vi "rx QAM.vi"() -> ()   [LabVIEW 2026]
uses:
  <instrlib>/niUSRP/niUSRP Fetch Rx Data (CDB Cluster).vi
  <vilib>/addons/Modulation/Digital/Demodulation/MT Calculate BER After Trigger (User Pattern).vi
  <vilib>/addons/Modulation/niDMT.lvlib
panel:
  in  "device names":refnum<k15>
  in  "pulse shaping filter (none)":T1(ring)=enum."Raised Cosine"
  out "Constellation Graph":T2(graph)
  out "BER":dbl=1.0 format="%.4f"
  out "output bit stream":i8[](array[numeric])
  in  "carrier frequency":dbl=434000000.0 format="%#_6p"
  in  "Rx IQ rate":dbl=400000.0
  in  "number of samples":i64=16536
  in  "Stop":bool
  out "Waveform Graph":dbl[][](graph)
  out "error out":errorcluster
  out "coerced gain":dbl format="%#_6f"
  out "coerced carrier frequency":dbl=1000000000.0 format="%#_6p"
  out "coerced IQ rate":dbl=400000.0 format="%.6p"
  in  "active antenna":string="RX2"
  in  "rx gain":dbl=20.0 format="%#_6f"
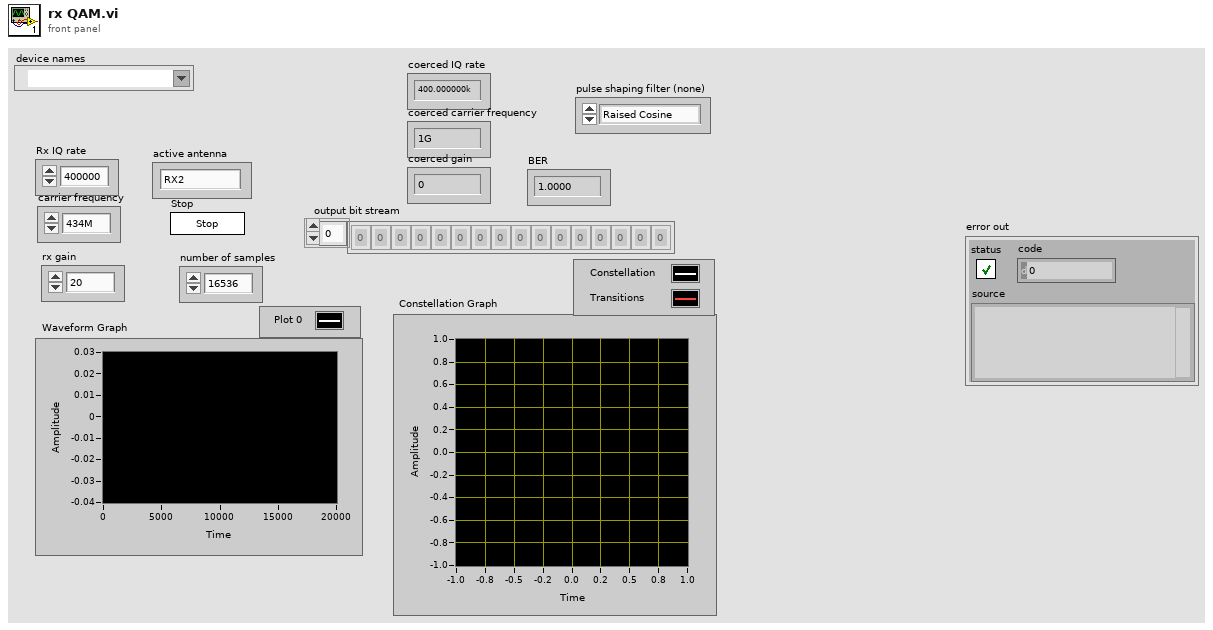
[diagram p1: front panel]
types:
  T1 = enum16{"none", "Raised Cosine", "Root Raised Cos", "Gaussian"}
  T2 = cluster{"constellation":dbl[], "oversampled data":dbl[]}[]
  T3 = cluster{"expected sync location (symbols)":i32, "sync sequence":cdb[], "sync location uncertainty (symbols)":i32, "sync indent (symbols)":i32}
  T4 = cluster{"samples per symbol (16)":i32, "symbol map":cdb[]}
  T5 = typedef "niAMT.lvlib/Complex Data Waveform.ctl" = cluster{"t0":dbl, "dt":dbl, "Y":cdb[]}
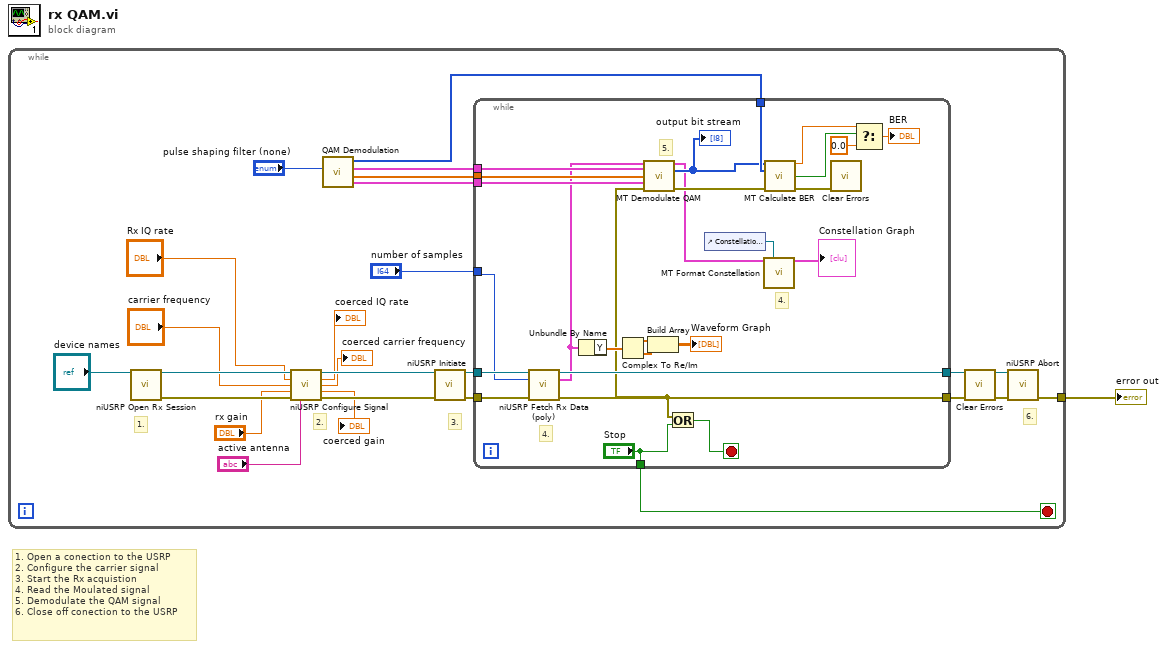
[diagram p0: block diagram]
diagram:
  # "1. Open a conection to the USRP\n2. Configure the carrier signal\n3. Start the Rx acquistion\n4. Read the Moulated signal\n5. Demodulate the QAM signal\n6. Close off conection to the USRP"
  n1 = while {
    tunnel: [w17] -> w1
    stop <- w8 stop-if-true
    # "6."
    # "3."
    # "2."
    # "1."
    n2 = call <instrlib>:"niUSRP Open Rx Session.vi"("device names"="device names") -> ("session handle out"=w26:refnum<k15>, "error out"=w25:errorcluster)  [unwired: 13 in]
    n3 = call <instrlib>:"niUSRP Configure Signal.vi"("session handle"=w26, "IQ rate"="Rx IQ rate", "carrier frequency"="carrier frequency", "gain"="rx gain", "error in (no error)"=w25, "active antenna"="active antenna") -> ("session handle out"=w21:refnum<k15>, "coerced IQ rate"=→"coerced IQ rate":dbl, "coerced carrier frequency"=→"coerced carrier frequency":dbl, "coerced gain"=→"coerced gain":dbl, "error out"=w22:errorcluster)  [unwired: 5 in]
    n4 = call "QAM Demodulation.vi"("pulse shaping filter (none)"="pulse shaping filter (none)") -> ("QAM synchronization parameters"=w5:T3, "matched filter coefficients"=w6:dbl[], "QAM system parameters"=w7:T4, "output bit stream"=w4:i8[])  [unwired: 6 in]
    n5 = call <instrlib>:"niUSRP Initiate.vi"("session handle"=w21, "error in (no error)"=w22) -> ("session handle out"=w14:refnum<k15>, "error out"=w13:errorcluster)  [unwired: 12 in]
    n6 = while {
      tunnel: w14 -> [w52]
      tunnel: w13 -> [w51]
      tunnel: [w50] -> w12
      tunnel: [w39] -> w11
      tunnel: "number of samples" -> [w35]
      tunnel: ["Stop"] -> w8
      tunnel: w7 -> [w43]
      tunnel: w6 -> [w42]
      tunnel: w5 -> [w41]
      tunnel: w4 -> [w40]
      stop <- w46 stop-if-true
      # "4."
      # "4."
      # "5."
      n7 = call-poly <instrlib>:"niUSRP Fetch Rx Data (poly).vi"("session handle"=w52, "number of samples"=w35, "error in (no error)"=w51) -> ("session handle out"=w50:refnum<k15>, "data"=w31:cluster{"t0":dbl, "dt":dbl, "Y":cdb[]}, "error out"=w39:errorcluster)  [unwired: 9 in, 1 out]
      n8 = Unbundle By Name(w31) -> ("Y"=w44:cdb[])
      n9 = Complex To Re/Im(x + iy=w44) -> (x=w47:dbl[], y=w49:dbl[])
      n10 = call <vilib>:"MT Demodulate QAM.vi"("input complex waveform"=w31, "QAM system parameters"=w43, "matched filter coefficients"=w42, "synchronization parameters"=w41, "error in (no error)"=w39) -> ("recovered complex waveform"=w32:T5, "output bit stream"=w33:i8[], "error out"=w34:errorcluster)  [unwired: 6 in, 2 out]
      "output bit stream" <- w33
      n11 = Build Array(w47, w49) -> (→"Waveform Graph":dbl[][])
      n12 = Or(x=w39, y="Stop") -> (x .or. y?=w46:bool)
      n13 = control-ref of="Constellation Graph"() -> (w37:refnum<vi>)
      n14 = call <vilib>:"MT Format Constellation.vi"("waveform"=w32, "constellation reference"=w37) -> ("constellation graph"=→"Constellation Graph":T2)  [unwired: 3 in, 10 out]
      n15 = call-poly <vilib>:"MT Calculate BER.vi"("input bit stream"=w33, "reference bit pattern"=w40, "error in (no error)"=w34) -> ("BER"=w29:dbl, "trigger found?"=w30:bool, "error out"=w36:errorcluster)  [unwired: 8 in, 2 out]
      n16 = call <vilib>:"Clear Errors.vi"("error in (no error)"=w36) -> ()  [unwired: 5 in, 2 out]
      n17 = Select(t=w29, s=w30, f=0.0) -> (s? t:f=→"BER":dbl)
    }
    n18 = call <vilib>:"Clear Errors.vi"("error in (no error)"=w11) -> ("error out"=w9:errorcluster)  [unwired: 5 in, 1 out]
    n19 = call <instrlib>:"niUSRP Abort.vi"("session handle"=w12, "error in (no error)"=w9) -> ("error out"=w17:errorcluster)  [unwired: 12 in, 1 out]
  }
  "error out" <- w1
